vi "Functional Global.vi"(7 "명령":T1, 8 "에러 입력 (에러 없음)":errorcluster caption="에러 입력(에러 없음)") -> (0 "에러 출력":errorcluster, 2 "카운트":i32)   [LabVIEW 2010]
uses:
  Functional Global Command.ctl
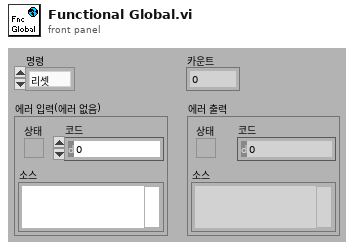
[diagram p1: front panel]
types:
  T1 = typedef "Functional Global Command.ctl" = enum16{"리셋", "증가", "카운트 가져오기"}
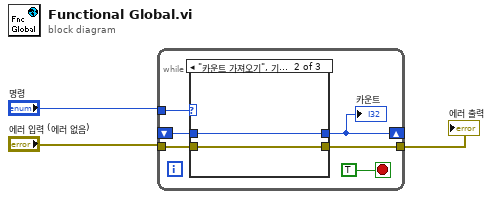
[diagram p0: block diagram]
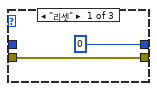
[diagram p2: hidden frame]
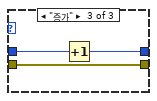
[diagram p3: hidden frame]
diagram:
  n1 = while {
    tunnel: "명령" -> [w8]
    shift-right: [w6] -> _
    shift-left: _ -> [w7]
    tunnel: "에러 입력 (에러 없음)" -> [w5]
    tunnel: [w4] -> w1
    stop <- TRUE stop-if-true
    n2 = case shown="\"카운트 가져오기\", 기본" w8 {
      tunnel: [0 w13 w15] -> w6
      tunnel: w7 -> [_ w13 w16]
      tunnel: [w10 w12 w14] -> w4
      tunnel: w5 -> [w10 w12 w14]
      frame "리셋" {
      }
      frame "카운트 가져오기", Default {
      }
      frame "증가" {
        n3 = Increment(x=w16) -> (x+1=w15:i32)
      }
    }
    "카운트" <- w6
  }
  "에러 출력" <- w1
